vi "DAQ_Task.vi"() -> (2 "输出簇":T1)   [LabVIEW 2016]
uses:
  <vilib>/DAQmx/create/channels.llb/DAQmx Create Channel (AO-Voltage-Basic).vi
  <vilib>/DAQmx/create/channels.llb/DAQmx Create Channel (AI-Voltage-Basic).vi
  <vilib>/DAQmx/create/channels.llb/DAQmx Create Channel (DO-Digital Output).vi
  <vilib>/DAQmx/create/channels.llb/DAQmx Create Channel (DI-Digital Input).vi
  <vilib>/DAQmx/create/channels.llb/DAQmx Create Channel (CO-Pulse Generation-Frequency).vi
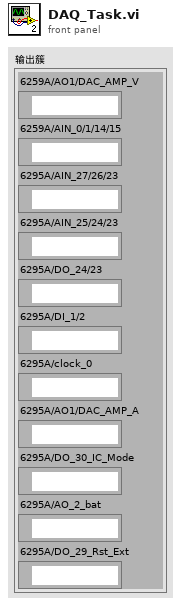
[diagram p1: front panel]
types:
  T1 = cluster{"6259A/AO1/DAC_AMP_V":refnum<k21>, "6259A/AIN_0/1/14/15":refnum<k21>, "6295A/AIN_27/26/23":refnum<k21>, "6295A/AIN_25/24/23":refnum<k21>, "6295A/DO_24/23":refnum<k21>, "6295A/DI_1/2":refnum<k21>, "6295A/clock_0":refnum<k21>, "6295A/AO1/DAC_AMP_A":refnum<k21>, "6295A/DO_30_IC_Mode":refnum<k21>, "6295A/AO_2_bat":refnum<k21>, "6295A/DO_29_Rst_Ext":refnum<k21>}
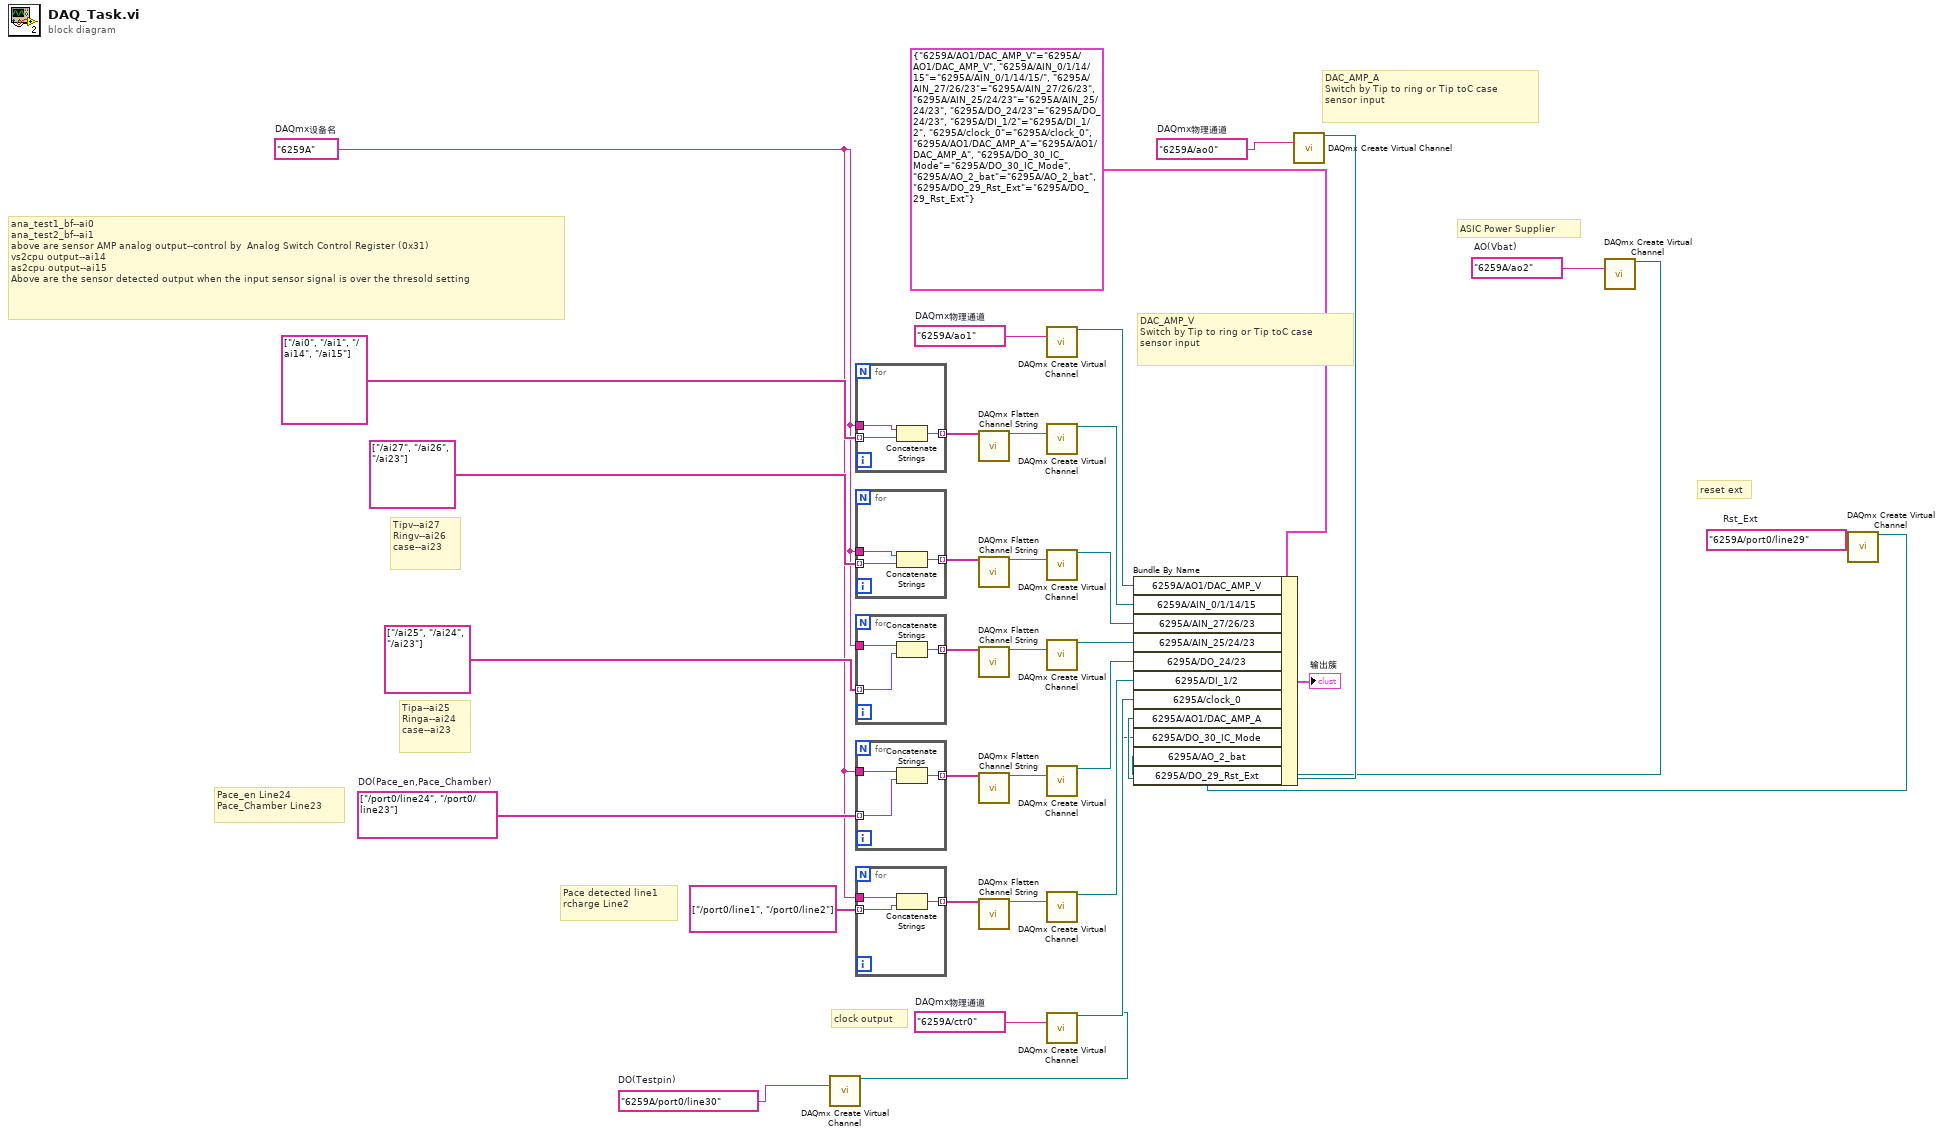
[diagram p0: block diagram]
diagram:
  w3 = tag "6259A/port0/line29"  # Rst_Ext
  w5 = tag "6259A/ao2"  # AO(Vbat)
  w7 = tag "6259A/port0/line30"  # DO(Testpin)
  w9 = tag "6259A/ao0"  # DAQmx物理通道
  w11 = tag "6259A/ctr0"  # DAQmx物理通道
  w20 = string[] ["/port0/line24", "/port0/line23"]  # DO(Pace_en,Pace_Chamber)
  w14 = tag "6259A"  # DAQmx设备名
  w35 = tag "6259A/ao1"  # DAQmx物理通道
  # "reset ext"
  # "ASIC Power Supplier"
  # "DAC_AMP_A\nSwitch by Tip to ring or Tip toC case\nsensor input"
  # "clock output"
  # "Pace detected line1\nrcharge Line2"
  # "Pace_en Line24\nPace_Chamber Line23"
  # "Tipa--ai25\nRinga--ai24\ncase--ai23"
  # "Tipv--ai27\nRingv--ai26\ncase--ai23"
  # "ana_test1_bf--ai0\nana_test2_bf--ai1\nabove are sensor AMP analog output--control by \tAnalog Switch Control Register (0x31)  \nvs2cpu output--ai14\nas2cpu output--ai15\nAbove are the sensor detected output when the input sensor signal is over the thresold setting"
  # "DAC_AMP_V\nSwitch by Tip to ring or Tip toC case\nsensor input"
  n1 = call-poly <vilib>:"DAQmx Create Virtual Channel.vi"("lines"=w7) -> ("task out"=w6:refnum<k21>)  [unwired: 13 in, 1 out]
  n2 = for {
    tunnel: string[] ["/ai0", "/ai1", "/ai14", "/ai15"] -> [w38] mode=indexing
    tunnel: w14 -> [w37]
    tunnel: [w36] -> w33 mode=indexing
    n3 = Concatenate Strings(w37, w38) -> (w36:string)
  }
  n4 = for {
    tunnel: string[] ["/ai27", "/ai26", "/ai23"] -> [w41] mode=indexing
    tunnel: w14 -> [w40]
    tunnel: [w39] -> w26 mode=indexing
    n5 = Concatenate Strings(w40, w41) -> (w39:string)
  }
  n6 = for {
    tunnel: string[] ["/ai25", "/ai24", "/ai23"] -> [w44] mode=indexing
    tunnel: w14 -> [w43]
    tunnel: [w42] -> w22 mode=indexing
    n7 = Concatenate Strings(w43, w44) -> (w42:string)
  }
  n8 = for {
    tunnel: w20 -> [w47] mode=indexing
    tunnel: w14 -> [w46]
    tunnel: [w45] -> w19 mode=indexing
    n9 = Concatenate Strings(w46, w47) -> (w45:string)
  }
  n10 = for {
    tunnel: string[] ["/port0/line1", "/port0/line2"] -> [w50] mode=indexing
    tunnel: w14 -> [w49]
    tunnel: [w48] -> w15 mode=indexing
    n11 = Concatenate Strings(w49, w50) -> (w48:string)
  }
  n12 = call <vilib>:"DAQmx Flatten Channel String.vi"("names in"=w33) -> ("names out"=w29:string)  [unwired: 13 in, 1 out]
  n13 = call <vilib>:"DAQmx Flatten Channel String.vi"("names in"=w26) -> ("names out"=w27:string)  [unwired: 13 in, 1 out]
  n14 = call <vilib>:"DAQmx Flatten Channel String.vi"("names in"=w22) -> ("names out"=w23:string)  [unwired: 13 in, 1 out]
  n15 = call <vilib>:"DAQmx Flatten Channel String.vi"("names in"=w19) -> ("names out"=w18:string)  [unwired: 13 in, 1 out]
  n16 = call <vilib>:"DAQmx Flatten Channel String.vi"("names in"=w15) -> ("names out"=w16:string)  [unwired: 13 in, 1 out]
  n17 = call-poly <vilib>:"DAQmx Create Virtual Channel.vi"("physical channels"=w35) -> ("task out"=w32:refnum<k21>)  [unwired: 13 in, 1 out]
  n18 = call-poly <vilib>:"DAQmx Create Virtual Channel.vi"("physical channels"=w29) -> ("task out"=w30:refnum<k21>)  [unwired: 13 in, 1 out]
  n19 = call-poly <vilib>:"DAQmx Create Virtual Channel.vi"("physical channels"=w27) -> ("task out"=w25:refnum<k21>)  [unwired: 13 in, 1 out]
  n20 = call-poly <vilib>:"DAQmx Create Virtual Channel.vi"("physical channels"=w23) -> ("task out"=w21:refnum<k21>)  [unwired: 13 in, 1 out]
  n21 = call-poly <vilib>:"DAQmx Create Virtual Channel.vi"("lines"=w18) -> ("task out"=w17:refnum<k21>)  [unwired: 13 in, 1 out]
  n22 = call-poly <vilib>:"DAQmx Create Virtual Channel.vi"("lines"=w16) -> ("task out"=w12:refnum<k21>)  [unwired: 13 in, 1 out]
  n23 = call-poly <vilib>:"DAQmx Create Virtual Channel.vi"("counter"=w11) -> ("task out"=w10:refnum<k21>)  [unwired: 13 in, 1 out]
  n24 = call-poly <vilib>:"DAQmx Create Virtual Channel.vi"("physical channels"=w9) -> ("task out"=w8:refnum<k21>)  [unwired: 13 in, 1 out]
  n25 = call-poly <vilib>:"DAQmx Create Virtual Channel.vi"("physical channels"=w5) -> ("task out"=w4:refnum<k21>)  [unwired: 13 in, 1 out]
  n26 = call-poly <vilib>:"DAQmx Create Virtual Channel.vi"("lines"=w3) -> ("task out"=w2:refnum<k21>)  [unwired: 13 in, 1 out]
  n27 = Bundle By Name(cluster=T1 {"6259A/AO1/DAC_AMP_V"="6295A/AO1/DAC_AMP_V", "6259A/AIN_0/1/14/15"="6295A/AIN_0/1/14/15/", "6295A/AIN_27/26/23"="6295A/AIN_27/26/23", "6295A/AIN_25/24/23"="6295A/AIN_25/24/23", "6295A/DO_24/23"="6295A/DO_24/23", "6295A/DI_1/2"="6295A/DI_1/2", "6295A/clock_0"="6295A/clock_0", "6295A/AO1/DAC_AMP_A"="6295A/AO1/DAC_AMP_A", "6295A/DO_30_IC_Mode"="6295A/DO_30_IC_Mode", "6295A/AO_2_bat"="6295A/AO_2_bat", "6295A/DO_29_Rst_Ext"="6295A/DO_29_Rst_Ext"}, "6259A/AO1/DAC_AMP_V"=w32, "6259A/AIN_0/1/14/15"=w30, "6295A/AIN_27/26/23"=w25, "6295A/AIN_25/24/23"=w21, "6295A/DO_24/23"=w17, "6295A/DI_1/2"=w12, "6295A/clock_0"=w10, "6295A/AO1/DAC_AMP_A"=w8, "6295A/DO_30_IC_Mode"=w6, "6295A/AO_2_bat"=w4, "6295A/DO_29_Rst_Ext"=w2) -> (→"输出簇":T1)
